vi "Intake Shooter Controller.vi"(8 "error in":errorcluster) -> ()   [LabVIEW 2019]
doc: "This VI executes continuously carrying out the current operation and responding to updates or new operations. It will often contain the timing or control code that is difficult to place directly in TeleOp. This VI generally opens all sensors and motors and isolates the rest of the robot code from knowing how the operations are carried out."
uses:
  <vilib>/Rock Robotics/WPI/Framework/Completion Status.ctl
  Intake Shooter Setpoints.ctl
  Intake Shooter Operations.ctl
  <vilib>/Rock Robotics/WPI/ThirdParty/REV Robotics/SPARK MAX/Typedef/Spark MAX Control Type.ctl
  <vilib>/Rock Robotics/Network Tables/NT Write Boolean.vi
panel:
  out "Iterations 3":i32
  out "Analog Position 2":dbl
  out "Iterations 2":i32
  out "Iterations":i32
  out "Analog Position":dbl
  in  "Interactive Values":T1
  out "Current\nCmd":string
  in  "Buttons":cluster{"Execute Cmd":bool, "Abort Cmd":bool}
  out "Command Timing":cluster{"Start Time (ms)":u32, "Iterations":i32}
  out "Status":T3
  # "Tip: It may be helpful to observe inputs and sensor values.\nYou may also want to display tuning or debugging controls."
  # "Interactive Command: You may fill in the settings for a command\nand schedule it with the Execute button. You can observe and abort\nany command while fine tuning the code for the controller."
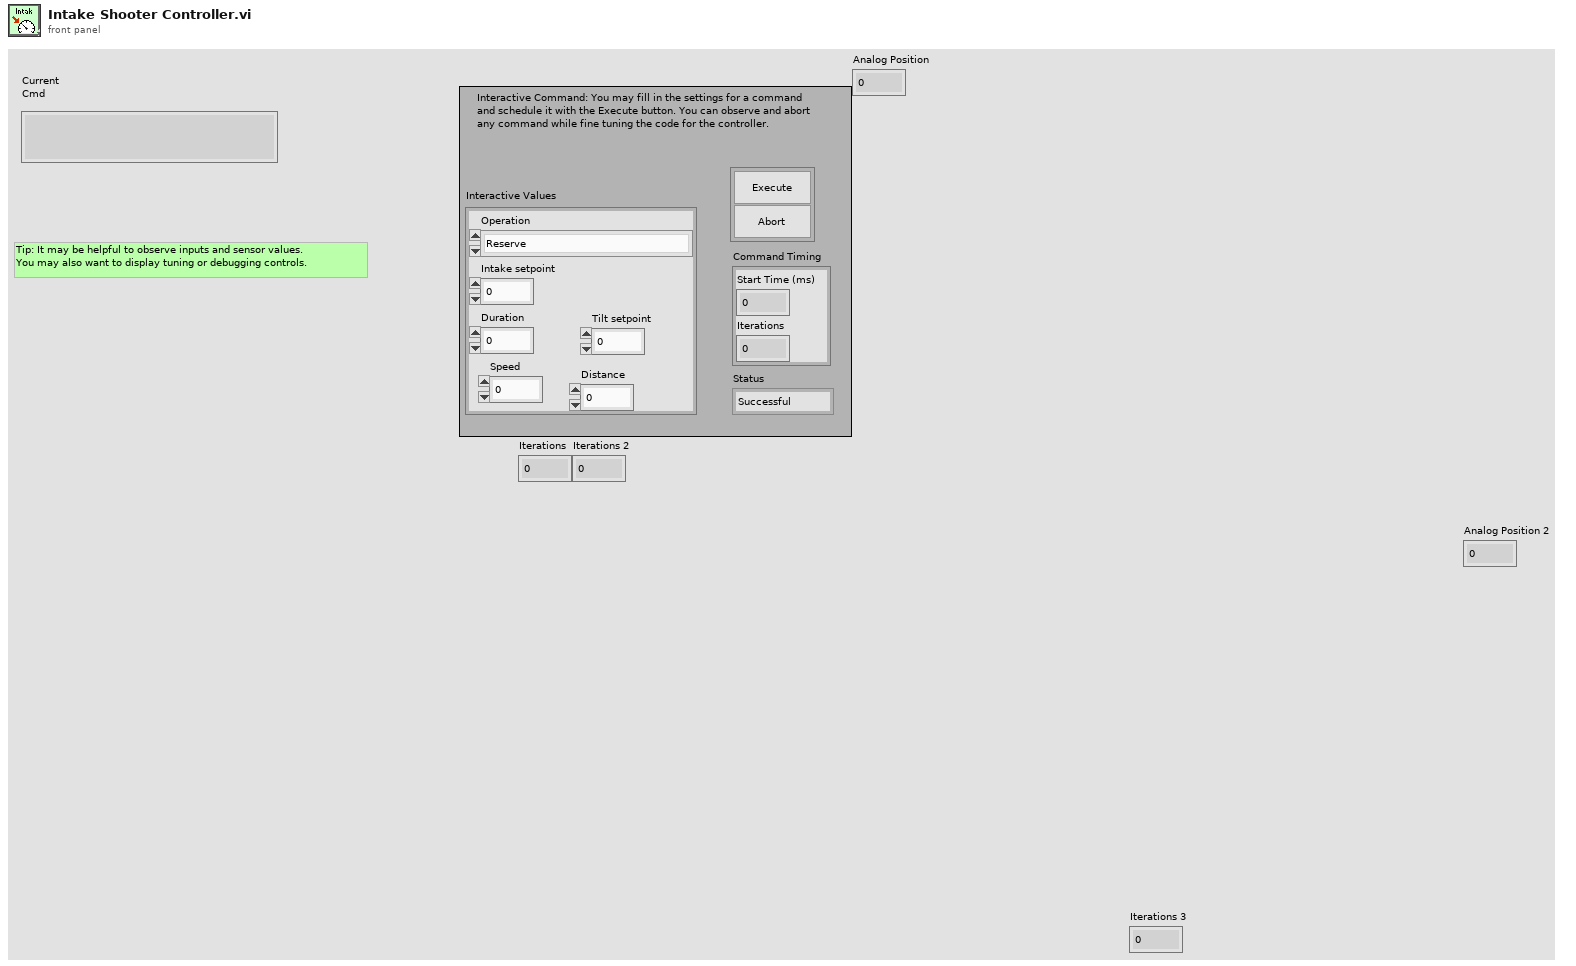
[diagram p1: front panel]
types:
  T1 = typedef "Intake Shooter Setpoints.ctl" = cluster{"Operation":T2, "Intake setpoint":dbl, "Duration":dbl, "Tilt setpoint":dbl, "Speed":dbl, "Distance":dbl}
  T2 = typedef "Intake Shooter Operations.ctl" = enum16{"Reserve", "Read Current", "Immediate", "Go up", "Go down", "Armediate"}
  T3 = typedef "Completion Status.ctl" = enum16{"Successful", "Aborted", "Incomplete"}
  T4 = typedef "WPI_MotorControlDeviceRef.ctl" = cluster{"DeviceStatus":errorcluster, "Type":T5, "PWM":cluster{"PWM Channel":T6, "DeadBand":T7}, "CAN":cluster{"Device Number":u8, "SetOutput VI Ref":variant, "GetOutput VI Ref":variant, "Enable VI Ref":variant, "Disable VI Ref":variant, "Data":variant}, "Invert":bool, "DIO PWM":cluster{"PWM \"Enable\" Channel":T6, "DIOChannel":T8, "PWM Rate":dbl}}
  T5 = typedef "WPI_MotorControlType.ctl" = enum16{"PWM", "CAN", "DIO PWM"}
  T6 = typedef "FPGA_DIOPWMChannel.ctl" = enum8{"PWM 0", "PWM 1", "PWM 2", "PWM 3", "PWM 4", "PWM 5", "PWM 6", "PWM 7", "PWM 8", "PWM 9", "PWM MXP 0", "PWM MXP 1", "PWM MXP 2", "PWM MXP 3", "PWM MXP 4", "PWM MXP 5", "PWM MXP 6", "PWM MXP 7", "PWM MXP 8", "PWM MXP 9", "Invalid"}
  T7 = typedef "WPI_PWMDeadband.ctl" = cluster{"Name":string, "maxPositivePwm":i32, "minPositivePwm":i32, "centerPwm":i32, "maxNegativePwm":i32, "minNegativePwm":i32, "angularRange":u16}
  T8 = typedef "FPGA_DIOChannel.ctl" = enum8{"DIO 0", "DIO 1", "DIO 2", "DIO 3", "DIO 4", "DIO 5", "DIO 6", "DIO 7", "DIO 8", "DIO 9", "DIO MXP 0", "DIO MXP 1", "DIO MXP 2", "DIO MXP 3", "DIO MXP 4", "DIO MXP 5", "DIO MXP 6", "DIO MXP 7", "DIO MXP 8", "DIO MXP 9", "DIO MXP 10", "DIO MXP 11", "DIO MXP 12", "DIO MXP 13", "DIO MXP 14", "DIO MXP 15", "SPI Port CS1", "SPI Port CS2", "SPI Port CS3", "SPI Port MISO", "SPI Port MOSI", "Invalid"}
  T9 = typedef "Command Status Info.ctl" = cluster{"Name":string, "Status":T3, "notifier out":T10}
  T10 = typedef "Completion Notifier.ctl" = refnum<notifier>
  T11 = cluster{"Current Command":T1, "Command Timing":cluster{"Start Time (ms)":u32, "Iterations":i32}, "Command Arguments":cluster{"Command Info":T9, "Description":string, "Default Command":T1, "queue out":refnum<queue>, "Subsystem Name":string}}
  T12 = typedef "Spark MAX Control Type.ctl" = enum16{"Percent VBus", "Voltage", "Velocity", "Position", "Smart Motion", "Current", "Smart Velocity"}
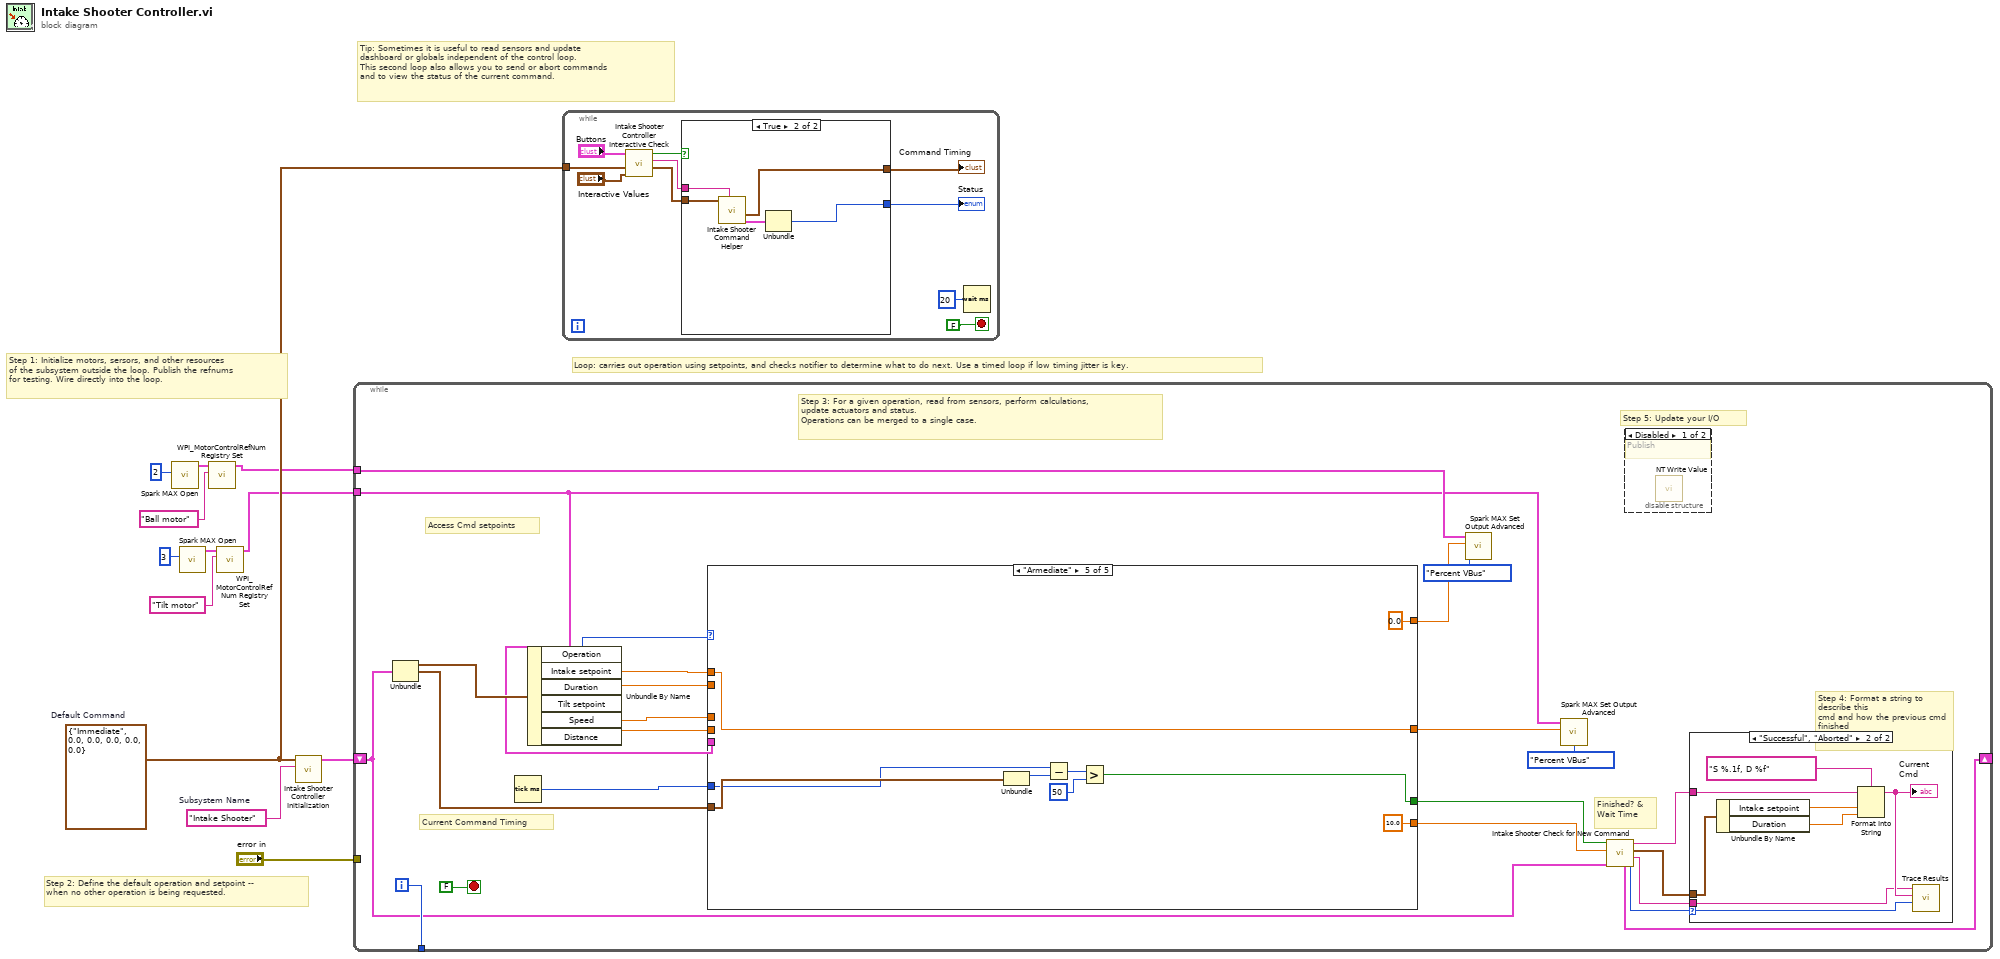
[diagram p0: block diagram]
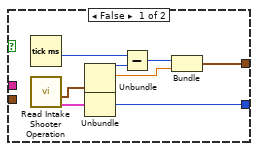
[diagram p2: hidden frame]
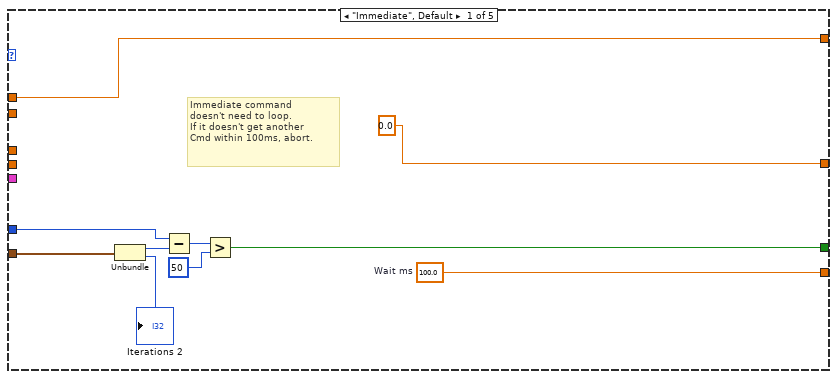
[diagram p4: hidden frame]
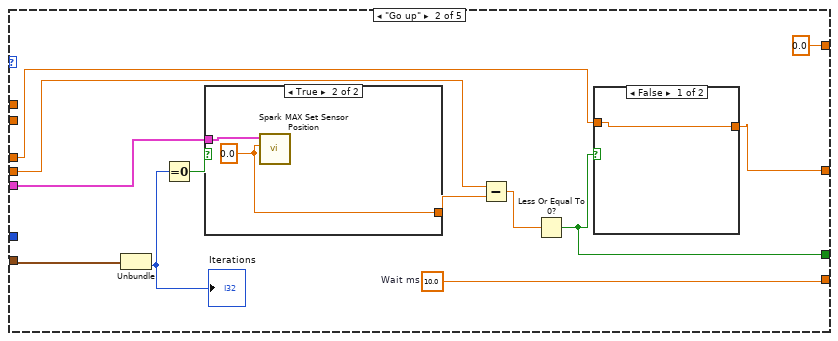
[diagram p5: hidden frame]
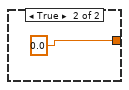
[diagram p6: hidden frame]
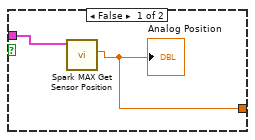
[diagram p7: hidden frame]
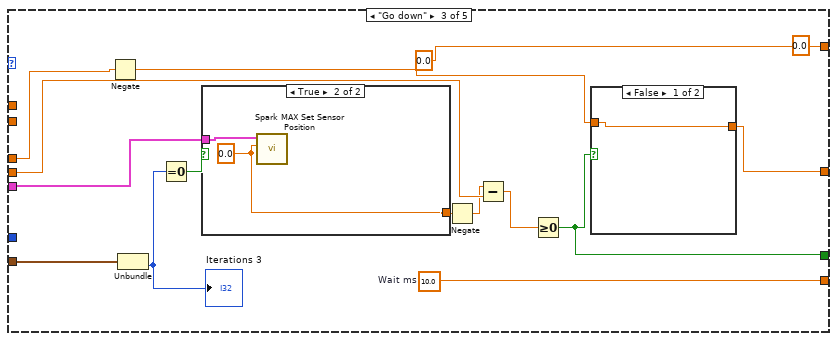
[diagram p8: hidden frame]
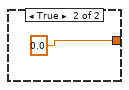
[diagram p9: hidden frame]
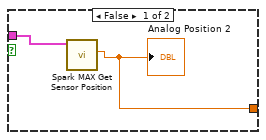
[diagram p10: hidden frame]
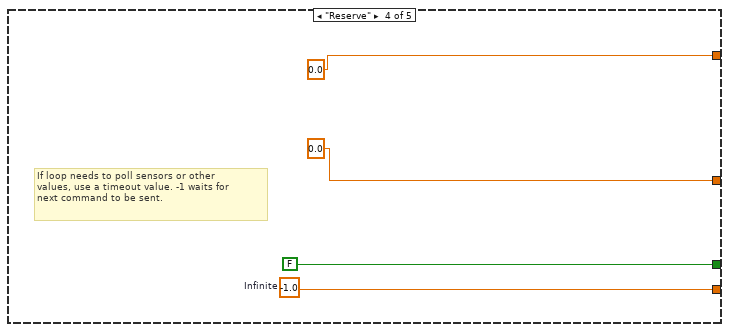
[diagram p11: hidden frame]
diagram:
  w9 = T1 {"Operation"=enum."Immediate", "Intake setpoint"=0.0, "Duration"=0.0, "Tilt setpoint"=0.0, "Speed"=0.0, "Distance"=0.0}  # Default Command
  w10 = "Intake Shooter"  # Subsystem Name
  # "Tip: Sometimes it is useful to read sensors and update\ndashboard or globals independent of the control loop.\nThis second loop also allows you to send or abort commands\nand to view the status of the current command."
  # "Step 2: Define the default operation and setpoint --\nwhen no other operation is being requested."
  # "Step 1: Initialize motors, sersors, and other resources\nof the subsystem outside the loop. Publish the refnums\nfor testing. Wire directly into the loop."
  # "Loop: carries out operation using setpoints, and checks notifier to determine what to do next. Use a timed loop if low timing jitter is key."
  n1 = call <vilib>:"Spark MAX Open.vi"("Device Number"=u8 2) -> ("MotorControlDeviceRef"=w3:T4)  [unwired: 9 in, 1 out]
  n2 = call <vilib>:"Spark MAX Open.vi"("Device Number"=u8 3) -> ("MotorControlDeviceRef"=w7:T4)  [unwired: 9 in, 1 out]
  n3 = call <vilib>:"WPI_MotorControlRefNum Registry Set.vi"("refnum name"="Ball motor", "MotorControlDevRef"=w3) -> ("MotorControlDevRef"=w1:T4)  [unwired: 8 in, 1 out]
  n4 = call <vilib>:"WPI_MotorControlRefNum Registry Set.vi"("refnum name"="Tilt motor", "MotorControlDevRef"=w7) -> ("MotorControlDevRef"=w5:T4)  [unwired: 8 in, 1 out]
  n5 = call "Intake Shooter Controller Initialization.vi"("Subsystem Name"=w10, "Default Command"=w9) -> ("Current Command"=w11:T11)  [unwired: 9 in]
  n6 = while {
    shift-right: [w29] -> _
    shift-left: w11 -> [w22]
    tunnel: [w35] -> _
    tunnel: "error in" -> [_]
    tunnel: w1 -> [w21]
    tunnel: w5 -> [w15]
    i -> [w35]
    stop <- FALSE stop-if-true
    # "Step 5: Update your I/O"
    # "Step 4: Format a string to describe this\ncmd and how the previous cmd finished"
    # "Current Command Timing"
    # "Access Cmd setpoints"
    # "Finished? &\nWait Time"
    # "Step 3: For a given operation, read from sensors, perform calculations,\nupdate actuators and status.\nOperations can be merged to a single case."
    n7 = Unbundle(w22) -> ("Current Command"=w34:T1, "Command Timing"=w31:cluster{"Start Time (ms)":u32, "Iterations":i32})  [unwired: 1 out]
    n8 = Tick Count (ms)() -> (millisecond timer value=w32:u32)
    n9 = Unbundle By Name(w34) -> ("Operation"=w33:T2, "Intake setpoint"=w30:dbl, "Duration"=w18:dbl, "Speed"=w17:dbl, "Distance"=w16:dbl)  [unwired: 1 out]
    n10 = case shown="\"Armediate\"" w33 {
      tunnel: [w46 w58 w69 w88 10.0 ("Infinite")] -> w27
      tunnel: [w40 w48 w70 FALSE ("ignore previous (F)") w91] -> w28
      tunnel: w31 -> [w42 w57 w68 _ w92]
      tunnel: w32 -> [w41 _ _ _ w90]
      tunnel: w30 -> [w39 _ _ _ w96]
      tunnel: [w39 0.0 ("f") 0.0 ("f") 0.0 ("f") 0.0 ("f")] -> w20
      tunnel: [0.0 ("Setpoint") w50 w71 0.0 w96] -> w19
      tunnel: w15 -> [_ w54 w74 _ _]
      tunnel: w18 -> [_ _ _ _ _]
      tunnel: w17 -> [_ w49 w73 _ _]
      tunnel: w16 -> [_ w53 w67 _ _]
      frame "Immediate", Default {
        w46 = 100.0  # Wait ms
        # "Immediate command\ndoesn't need to loop.\nIf it doesn't get another\nCmd within 100ms, abort."
        n11 = Unbundle(w42) -> ("Start Time (ms)"=w45:u32, "Iterations"=→"Iterations 2":i32)
        n12 = Subtract(x=w41, y=w45) -> (x-y=w44:u32)
        n13 = Greater?(x=w44, y=u8 50 ("Left Motor")) -> (0:w40:bool)
      }
      frame "Go up" {
        w58 = 10.0  # Wait ms
        n14 = Unbundle(w57) -> ("Iterations"=w56:i32)  [unwired: 1 out]
        "Iterations" <- w56
        n15 = Equal To 0?(x=w56) -> (x = 0?=w55:bool)
        n16 = case shown="True" w55 {
          tunnel: w54 -> [w61 w64]
          tunnel: [w62 w63] -> w52
          frame False {
            n17 = call <vilib>:"Spark MAX Get Sensor Position.vi"("MotorControlDevRef in"=w61) -> ("Sensor Position"=w62:dbl)  [unwired: 7 in, 3 out]
            "Analog Position" <- w62
          }
          frame True {
            w63 = 0.0 ("Position")
            n18 = call <vilib>:"Spark MAX Set Sensor Position.vi"("Position"=w63, "MotorControlDeviceRef"=w64) -> ()  [unwired: 8 in, 2 out]
          }
        }
        n19 = Subtract(x=w53, y=w52) -> (x-y=w51:dbl)
        n20 = Less Or Equal To 0?(x=w51) -> (x <= 0?=w48:bool)
        n21 = case shown="False" w48 {
          tunnel: [w59 0.0 ("Setpoint")] -> w50
          tunnel: w49 -> [w59 _]
          frame False {
          }
          frame True {
          }
        }
      }
      frame "Go down" {
        (unwired) 0.0 ("f")
        w69 = 10.0  # Wait ms
        n22 = Negate(x=w73) -> (-x=w72:dbl)
        n23 = Unbundle(w68) -> ("Iterations"=w77:i32)  [unwired: 1 out]
        "Iterations 3" <- w77
        n24 = Equal To 0?(x=w77) -> (x = 0?=w76:bool)
        n25 = case shown="True" w76 {
          tunnel: w74 -> [w81 w84]
          tunnel: [w82 w83] -> w66
          frame False {
            n26 = call <vilib>:"Spark MAX Get Sensor Position.vi"("MotorControlDevRef in"=w81) -> ("Sensor Position"=w82:dbl)  [unwired: 7 in, 3 out]
            "Analog Position 2" <- w82
          }
          frame True {
            w83 = 0.0 ("Position")
            n27 = call <vilib>:"Spark MAX Set Sensor Position.vi"("Position"=w83, "MotorControlDeviceRef"=w84) -> ()  [unwired: 8 in, 2 out]
          }
        }
        n28 = Negate(x=w66) -> (-x=w65:dbl)
        n29 = Subtract(x=w65, y=w67) -> (x-y=w75:dbl)
        n30 = Greater Or Equal To 0?(x=w75) -> (x >= 0?=w70:bool)
        n31 = case shown="False" w70 {
          tunnel: [w79 0.0 ("Setpoint")] -> w71
          tunnel: w72 -> [w79 _]
          frame False {
          }
          frame True {
          }
        }
      }
      frame "Reserve" {
        w88 = -1.0  # Infinite
        # "If loop needs to poll sensors or other\nvalues, use a timeout value. -1 waits for\nnext command to be sent."
      }
      frame "Armediate" {
        n32 = Unbundle(w92) -> ("Start Time (ms)"=w94:u32)  [unwired: 1 out]
        n33 = Subtract(x=w90, y=w94) -> (x-y=w95:u32)
        n34 = Greater?(x=w95, y=u8 50 ("Left Motor")) -> (0:w91:bool)
      }
    }
    n35 = call <vilib>:"Spark MAX Set Output Advanced.vi"("Control Mode"=Spark_MAX_Control_Type."Percent VBus", "Setpoint"=w20, "MotorControlDevRef"=w21) -> ()  [unwired: 7 in, 2 out]
    n36 = call <vilib>:"Spark MAX Set Output Advanced.vi"("Control Mode"=Spark_MAX_Control_Type."Percent VBus", "Setpoint"=w19, "MotorControlDevRef"=w15) -> ()  [unwired: 7 in, 2 out]
    n37 = call "Intake Shooter Check for New Command.vi"("Current Command"=w22, "Wait time (ms)"=w27, "Finished?"=w28) -> ("Completion"=w23:T3, "Subsystem Name"=w24:string, "Current Command"=w25:T1, "Initial Trace String"=w26:string, "NextCommand"=w29:T11)  [unwired: 4 in]
    n38 = disable-structure shown="Disabled" {
      frame Disabled {
        # "Publish"
        n39 = call-poly <vilib>:"NT Write Value.vi"() -> ()  [unwired: 11 in, 1 out]
      }
      frame Enabled {
      }
    }
    n40 = case shown="\"Successful\", \"Aborted\"" w23 {
      selector: w23 -> [_ w105]
      tunnel: w26 -> [_ w101]
      tunnel: w25 -> [_ w102]
      tunnel: w24 -> [_ w98]
      frame "Incomplete", Default {
        # "Continuing current command"
      }
      frame "Successful", "Aborted" {
        # "Report and setup for next command"
        n41 = Unbundle By Name(w102) -> ("Intake setpoint"=w104:dbl, "Duration"=w99:dbl)
        n42 = Format Into String(format string="S %.1f, D %f", initial string=w101, w104, w99) -> (resulting string=w100:string)  [unwired: 1 in, 1 out]
        "Current\nCmd" <- w100
        n43 = call <vilib>:"Trace Results.vi"("Status of previous command"=w105, "Description"=w100, "Subsystem"=w98) -> ()  [unwired: 9 in]
      }
    }
  }
  n44 = while {
    tunnel: w9 -> [w112]
    stop <- FALSE stop-if-true
    n45 = call "Intake Shooter Controller Interactive Check.vi"("Interactive Command in"="Interactive Values", "Default Command"=w112, "Buttons"="Buttons") -> ("Interactive Command out"=w109:T1, "Trace String"=w110:string, "Schedule"=w111:bool)  [unwired: 6 in]
    n46 = case shown="True" w111 {
      tunnel: [w123 w128] -> w108
      tunnel: w109 -> [_ w126]
      tunnel: [w119 w124] -> w107
      tunnel: w110 -> [_ w127]
      frame False {
        n47 = Tick Count (ms)() -> (millisecond timer value=w118:u32)
        n48 = call "Read Intake Shooter Operation.vi"() -> ("Command Info"=w116:T9, "SubSystem Data"=w117:T1)  [unwired: 9 in, 1 out]
        n49 = Unbundle(w117) -> ("Operation"=w122:T2, "Intake setpoint"=w120:dbl)  [unwired: 4 out]
        n50 = Unbundle(w116) -> ("Status"=w123:T3)  [unwired: 2 out]
        n51 = Subtract(x=w118, y=w122) -> (x-y=w121:u32)
        n52 = Bundle(w121, "Intake setpoint"=w120) -> (w119:cluster{u32, "Intake setpoint":dbl})  [unwired: 1 in]
      }
      frame True {
        n53 = call "Intake Shooter Command Helper.vi"("Description"=w127, "SubSystem Data"=w126) -> ("Command Info Out"=w125:T9, "Command Timing"=w124:cluster{"Start Time (ms)":u32, "Iterations":i32})  [unwired: 7 in, 1 out]
        n54 = Unbundle(w125) -> ("Status"=w128:T3)  [unwired: 2 out]
      }
    }
    "Status" <- w108
    "Command Timing" <- w107
    n55 = Wait (ms)(milliseconds to wait=u32 20) -> ()  [unwired: 1 out]
  }
